vi "act-0012-1-cor.vi"() -> ()   [LabVIEW 2010]
panel:
  in  "Délai en ms":dbl(slide) scale=0.0..10.0
  in  "stop":bool
  out "Historique":dbl(graph)
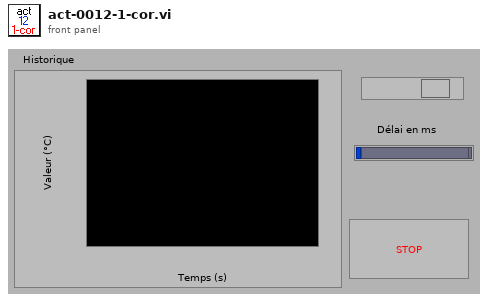
[diagram p1: front panel]
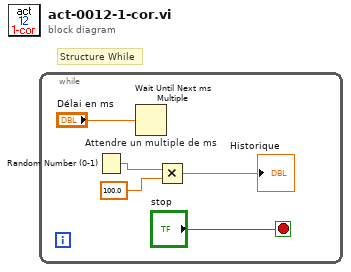
[diagram p0: block diagram]
diagram:
  # "Structure While"
  n1 = while {
    stop <- "stop" stop-if-true
    n2 = Random Number (0-1)() -> (number: 0 to 1=w4:dbl)
    n3 = Wait Until Next ms Multiple "Attendre un multiple de ms"(millisecond multiple="Délai en ms") -> ()  [unwired: 1 out]
    n4 = Multiply(x=w4, y=100.0) -> (x*y=→"Historique":dbl)
  }
